vi "Wrap Angle.vi"(1 "units":enum16{"degree", "radian", "gradian"}(ring), 2 "angle":dbl) -> (6 "wrapped angle":dbl)   [LabVIEW 2016]
doc: "Wraps an angle to be in the range of [ - 1/2 rotation, 1/2 rotation], where rotation is expressed in degrees, radians, or gradians. No unit conversion is performed."
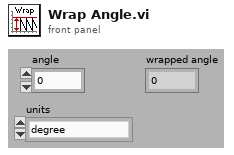
[diagram p1: front panel]
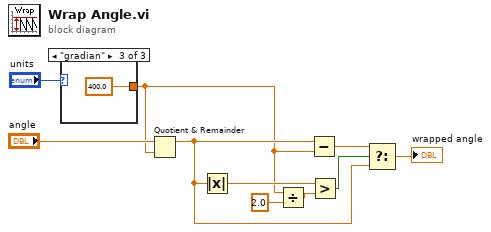
[diagram p0: block diagram]
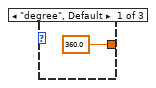
[diagram p2: hidden frame]
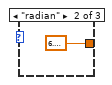
[diagram p3: hidden frame]
diagram:
  n1 = case shown="\"gradian\"" "units" {
    tunnel: [360.0 ("x") 6.283185307179586 400.0 ("x")] -> w2
    frame "degree", Default {
    }
    frame "radian" {
    }
    frame "gradian" {
    }
  }
  n2 = Quotient & Remainder(x="angle", y=w2) -> (x-y*floor(x/y)=w3:dbl)  [unwired: 1 out]
  n3 = Absolute Value(x=w3) -> (abs(x)=w10:dbl)
  n4 = Divide(x=w2, y=2.0) -> (x/y=w8:dbl)
  n5 = Subtract(x=w3, y=w2) -> (x-y=w1:dbl)
  n6 = Greater?(x=w10, y=w8) -> (0:w9:bool)
  n7 = Select(t=w1, s=w9, f=w3) -> (s? t:f=→"wrapped angle":dbl)
